vi "Check Execution Engine Connection.vi"(0 "message":string, 11 "error in (no error)":errorcluster) -> (15 "error out":errorcluster)   [LabVIEW 2023, in "RFCalAndFixtureCharact.Common.lvlib"]
uses:
  RFCalAndFixtureCharact.Common.lvlib
  C:/rfcal/AuxTools/STSRFFixtureCharactUtility/Source/Code Modules/Dependencies/NationalInstruments.RFCalibration.ExecutionEngine.dll
  Dependencies/NationalInstruments.RFCalibration.ExecutionEngine.dll
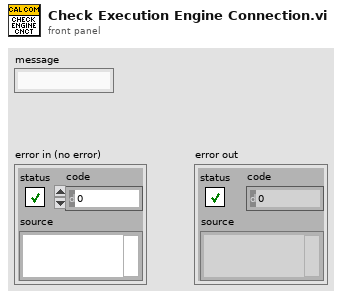
[diagram p1: front panel]
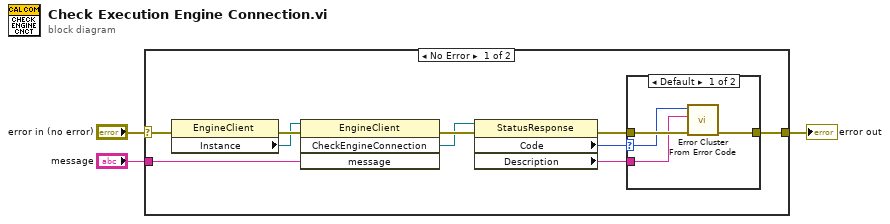
[diagram p0: block diagram]
diagram:
  n1 = case shown="No Error" "error in (no error)" {
    selector: "error in (no error)" -> [w12 w19]
    tunnel: [w6 w19] -> w2
    tunnel: "message" -> [w11 _]
    frame No Error {
      n2 = property class="EngineClient"(error in=w12) -> (error out=w10:errorcluster, "Instance"=w9:refnum<k24>)  [unwired: 1 in, 1 out]
      n3 = invoke class="EngineClient" method="CheckEngineConnection"(reference=w9, error in=w10, "message"=w11) -> (error out=w13:errorcluster, "CheckEngineConnection"=w4:refnum<k24>)  [unwired: 1 in, 2 out]
      n4 = property class="StatusResponse"(reference=w4, error in=w13) -> (error out=w7:errorcluster, "Code"=w8:i32, "Description"=w5:string)  [unwired: 1 out]
      n5 = case shown="Default" w8 {
        selector: w8 -> [w14 _]
        tunnel: [w16 w18] -> w6
        tunnel: w7 -> [w17 w18]
        tunnel: w5 -> [w15 _]
        frame Default {
          n6 = call <vilib>:"Error Cluster From Error Code.vi"("error in (no error)"=w17, "error message (\"\")"=w15, "error code (0)"=w14) -> ("error out"=w16:errorcluster)  [unwired: 6 in]
        }
        frame 0 {
        }
      }
    }
    frame Error {
    }
  }
  "error out" <- w2
